vi "Programmatically Find Zombies.vi"() -> ()   [LabVIEW 2017]
doc: "A demonstration of programmatically finding all graves that contain a zombie in a VI. A grave is a Diagram Disable Structure with a #RIP bookmark tag for a label (tombstone) and a zombie is when the legacy code frame (Corpse) has been enabled and the refactored code frame (Spirit) has been disabled. The Graveyard - Complex.vi example is used as a target VI and a simple UI is implemented to cycle through highlighting graves that only contain zombies in the target."
uses:
  Toolkit/Toolkit.lvlib
panel:
  in  "Stop Button":bool
  in  "Next Button":bool
  # "Overview: Demonstrates programmatically finding all zombies using the Graveyard - Complex.vi example as a target\nInstructions:\n1. Run the VI\n2. The Graveyard - Complex.vi's block diagram will be displayed automatically\n3. Repeatedly click the Next button to cycle through highlighting and selecting each grave that contains a zombie in the block diagram.\n4. Click the Stop button to stop the VI and close the Graveyard - Complex.vi example target."
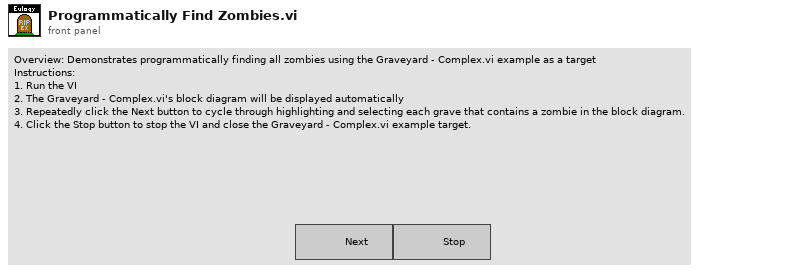
[diagram p1: front panel]
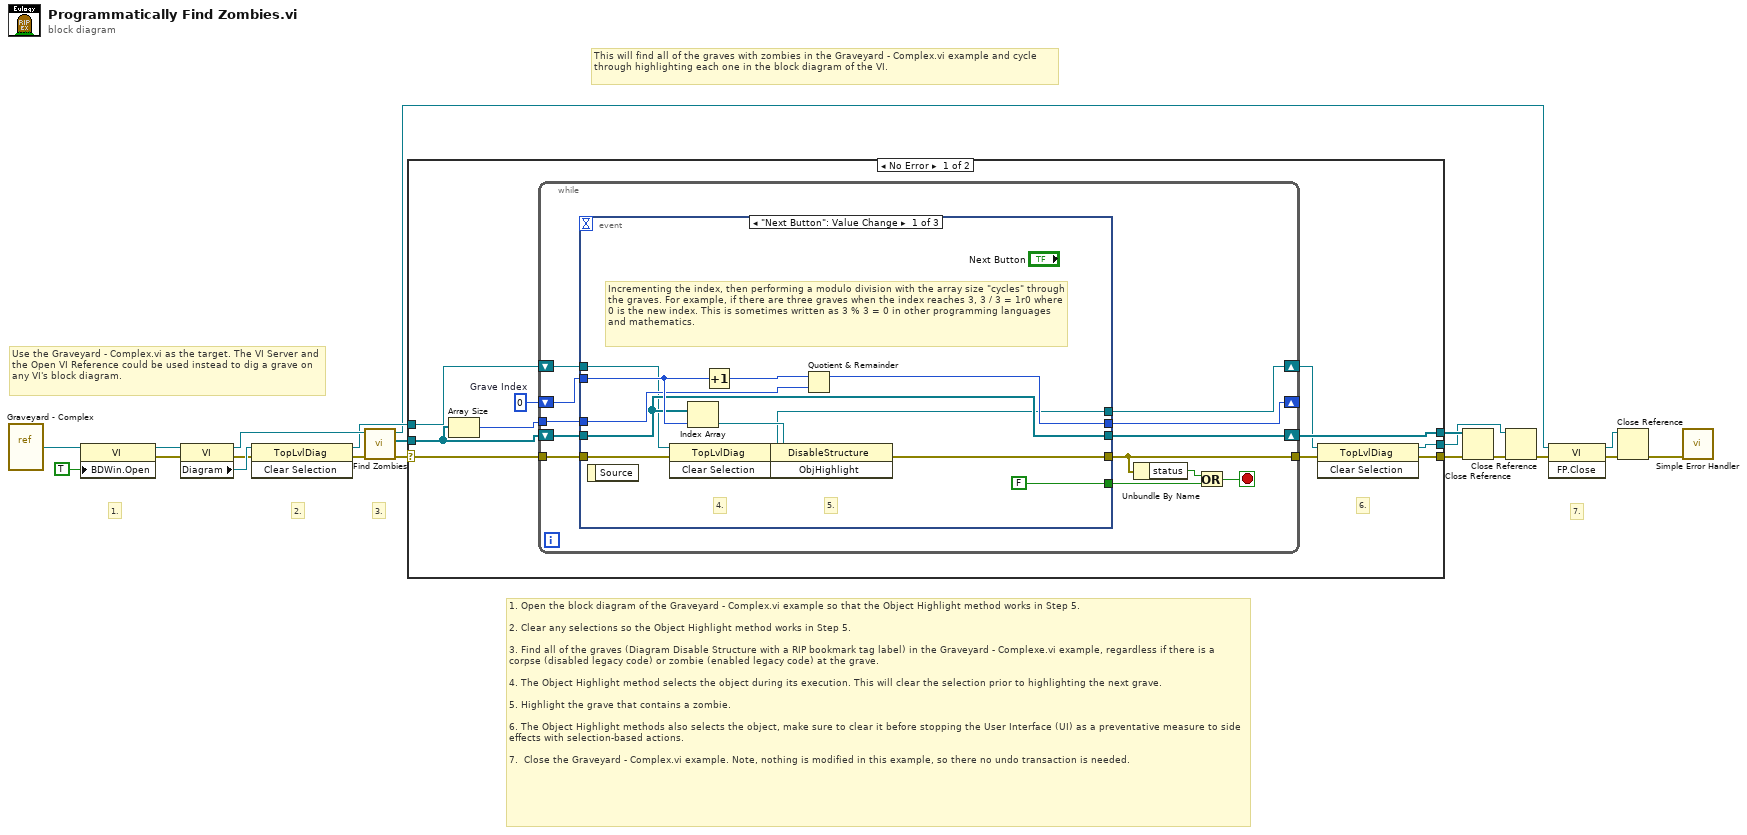
[diagram p0: block diagram]
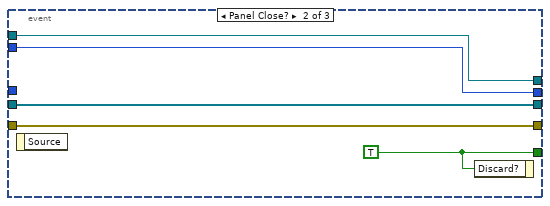
[diagram p2: hidden frame]
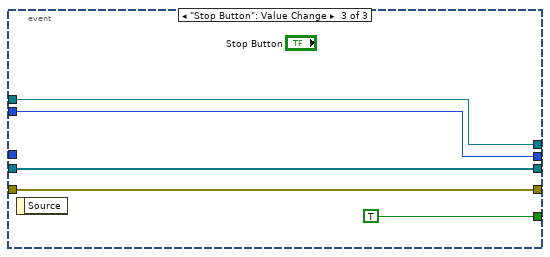
[diagram p3: hidden frame]
diagram:
  # "1. Open the block diagram of the Graveyard - Complex.vi example so that the Object Highlight method works in Step 5.\n\n2. Clear any selections so the Object Highlight method works in Step 5.\n\n3. Find all of the graves (Diagram Disable Structure with a RIP bookmark tag label) in the Graveyard - Complexe.vi example, regardless if there is a corpse (disabled legacy code) or zombie (enabled legacy code) at the grave.\n\n4. The Object Highlight method selects the object during its execution. This will clear the selection prior to highlighting the next grave.\n\n5. Highlight the grave that contains a zombie.\n\n6. The Object Highlight methods also selects the object, make sure to clear it before stopping the User Interface (UI) as a preventative measure to side effects with selection-based actions.\n\n7.  Close the Graveyard - Complex.vi example. Note, nothing is modified in this example, so there no undo transaction is needed."
  # "7."
  # "3."
  # "2."
  # "1."
  # "This will find all of the graves with zombies in the Graveyard - Complex.vi example and cycle through highlighting each one in the block diagram of the VI."
  # "Use the Graveyard - Complex.vi as the target. The VI Server and the Open VI Reference could be used instead to dig a grave on any VI's block diagram."
  n1 = vi-ref "Graveyard - Complex.vi"() -> (w16:refnum<vi>)
  n2 = property class="VI"(reference=w16, "BDWin.Open"=TRUE ("Block Diagram Window:Open")) -> (reference out=w13:refnum<vi>, error out=w12:errorcluster)  [unwired: 1 in]
  n3 = property class="VI"(reference=w13, error in=w12) -> (reference out=w10:refnum<vi>, error out=w14:errorcluster, "Diagram"=w15:refnum<vi>)
  n4 = invoke class="TopLvlDiag" method="Clear Selection"(reference=w15, error in=w14) -> (reference out=w9:refnum<vi>, error out=w11:errorcluster)  [unwired: 1 in, 1 out]
  n5 = call "Find Zombies.vi"("Error In"=w11, "VI In"=w10) -> ("Error Out"=w6:errorcluster, "Graves"=w20:refnum<vi>[], "VI Out"=w4:refnum<vi>)  [unwired: 7 in]
  n6 = case shown="No Error" w6 {
    selector: w6 -> [w27 w66]
    tunnel: w20 -> [w29 w67]
    tunnel: [w23 w66] -> w19
    tunnel: [w26 w67] -> w18
    tunnel: w9 -> [w25 w65]
    tunnel: [w21 w65] -> w7
    frame No Error {
      w30 = 0  # Grave Index
      # "6."
      n7 = Array Size(array=w29) -> (size(s)=w28:i32)
      n8 = while {
        shift-right: [w41] -> _
        shift-left: w30 -> [w42]
        shift-right: [w38] -> w26
        shift-left: w29 -> [w40]
        tunnel: w28 -> [w39]
        tunnel: w27 -> [w37]
        tunnel: [w36] -> w24
        shift-right: [w31] -> w22
        shift-left: w25 -> [w32]
        stop <- w34 stop-if-true
        n9 = event shown="[0] \"Next Button\": Value Change" {
          selector: _ -> [_ _ _]
          dyn-events: _ -> [_ _ _]
          timeout: _ -> [_ _ _]
          tunnel: w40 -> [w49 w59 w64]
          tunnel: w42 -> [w52 w56 w62]
          tunnel: [w53 w56 w62] -> w41
          tunnel: w39 -> [w50 _ _]
          tunnel: [w49 w59 w64] -> w38
          tunnel: w37 -> [w45 w57 w63]
          tunnel: [w48 w57 w63] -> w36
          tunnel: [FALSE w58 TRUE ("Discard?")] -> w33
          tunnel: w32 -> [w46 w55 w60]
          tunnel: [w43 w55 w60] -> w31
          event "Next Button": Value Change {
            # "Incrementing the index, then performing a modulo division with the array size \"cycles\" through the graves. For example, if there are three graves when the index reaches 3, 3 / 3 = 1r0 where 0 is the new index. This is sometimes written as 3 % 3 = 0 in other programming languages and mathematics."
            # "5."
            # "4."
            n10 = event-data() -> ()  [unwired: 1 in, 1 out]
            n11 = invoke class="TopLvlDiag" method="Clear Selection"(reference=w46, error in=w45) -> (reference out=w43:refnum<vi>, error out=w44:errorcluster)  [unwired: 1 in, 1 out]
            n12 = Index Array(array=w49, index=w52) -> (element=w51:refnum<vi>)
            n13 = Increment(x=w52) -> (x+1=w54:i32)
            n14 = invoke class="DisableStructure" method="ObjHighlight"(reference=w51, error in=w44) -> (error out=w48:errorcluster)  [unwired: 1 in, 2 out]
            n15 = Quotient & Remainder(x=w54, y=w50) -> (x-y*floor(x/y)=w53:i32)  [unwired: 1 out]
          }
          event Panel Close? {
            w58 = TRUE ("Discard?")
            n16 = event-data() -> ()  [unwired: 1 in, 1 out]
            n17 = event-data("Discard?"=w58) -> ()  [unwired: 1 in, 1 out]
          }
          event "Stop Button": Value Change {
            n18 = event-data() -> ()  [unwired: 1 in, 1 out]
          }
        }
        n19 = Unbundle By Name(w36) -> ("status"=w35:bool)
        n20 = Or(x=w35, y=w33) -> (x .or. y?=w34:bool)
      }
      n21 = invoke class="TopLvlDiag" method="Clear Selection"(reference=w22, error in=w24) -> (reference out=w21:refnum<vi>, error out=w23:errorcluster)  [unwired: 1 in, 1 out]
    }
    frame Error {
    }
  }
  n22 = Close Reference(reference=w18, error in (no error)=w19) -> (error out=w8:errorcluster)
  n23 = Close Reference(reference=w7, error in (no error)=w8) -> (error out=w5:errorcluster)
  n24 = invoke class="VI" method="FP.Close"(reference=w4, error in=w5) -> (reference out=w2:refnum<vi>, error out=w3:errorcluster)  [unwired: 1 in, 1 out]
  n25 = Close Reference(reference=w2, error in (no error)=w3) -> (error out=w1:errorcluster)
  n26 = call <vilib>:"Simple Error Handler.vi"("error in (no error)"=w1) -> ()  [unwired: 4 in, 5 out]
